vi "帧16打包.vi"(0 "帧ID":i8 format="%x", 4 "8":i16, 5 "1":i16, 6 "7":i16, 7 "2":i16, 8 "6":i16, 9 "5":i16, 10 "4":i16, 11 "3":i16) -> (3 "打包":string)   [LabVIEW 2016]
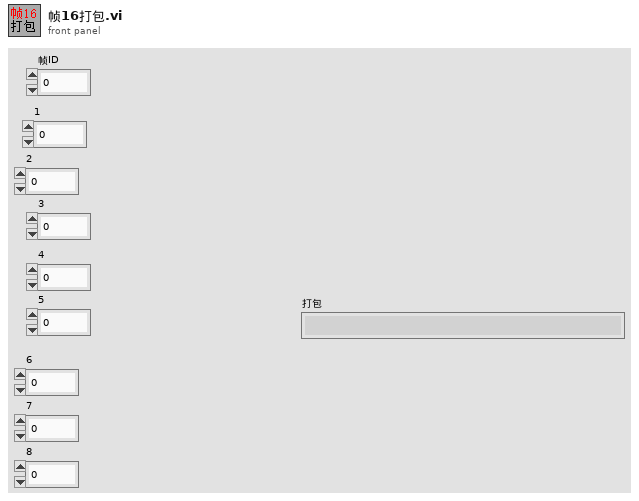
[diagram p1: front panel]
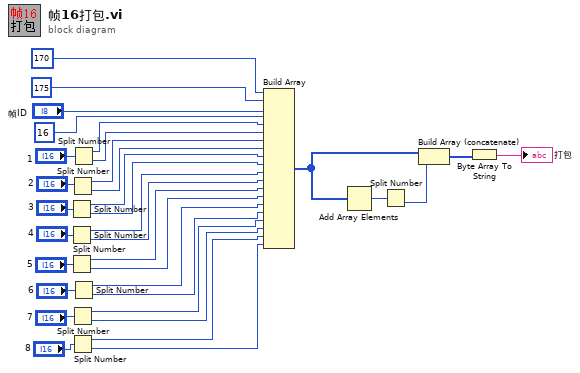
[diagram p0: block diagram]
diagram:
  n1 = Split Number(x="3") -> (hi(x)=w19:u8, lo(x)=w18:u8)
  n2 = Split Number(x="4") -> (hi(x)=w17:u8, lo(x)=w16:u8)
  n3 = Split Number(x="5") -> (hi(x)=w15:u8, lo(x)=w14:u8)
  n4 = Split Number(x="2") -> (hi(x)=w21:u8, lo(x)=w20:u8)
  n5 = Split Number(x="7") -> (hi(x)=w4:u8, lo(x)=w3:u8)
  n6 = Split Number(x="8") -> (hi(x)=w2:u8, lo(x)=w1:u8)
  n7 = Split Number(x="1") -> (hi(x)=w23:u8, lo(x)=w22:u8)
  n8 = Split Number(x="6") -> (hi(x)=w13:u8, lo(x)=w12:u8)
  n9 = Build Array(170, 175, "帧ID", i8 16, w23, w22, w21, w20, w19, w18, w17, w16, w15, w14, w13, w12, w4, w3, w2, w1) -> (w32:i32[])
  n10 = Add Array Elements(numeric array=w32) -> (sum=w33:i32)
  n11 = Split Number(x=w33) -> (lo(x)=w10:u16)  [unwired: 1 out]
  n12 = Build Array (concatenate)(w32, w10) -> (w31:i32[])
  n13 = Byte Array To String(unsigned byte array=w31) -> (string=→"打包":string)
